vi "lab2_new_p2.vi"() -> ()   [LabVIEW 2021]
panel:
  in  "x":dbl
  out "S":ext
  in  "n":u64
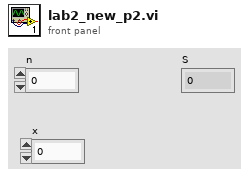
[diagram p1: front panel]
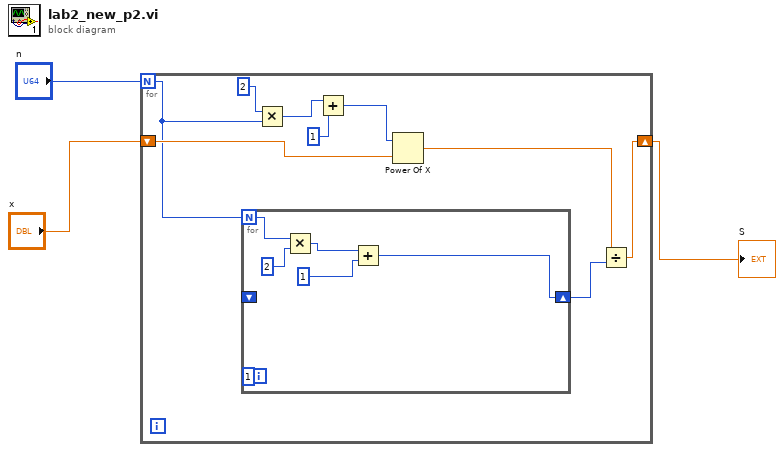
[diagram p0: block diagram]
diagram:
  n1 = for {
    N: "n" -> [w10]
    shift-right: [w4] -> w1
    shift-left: "x" -> [w12]
    n2 = for {
      N: w10 -> [w17]
      shift-right: [w13] -> w5
      shift-left: _ -> [_]
      (unwired) 1
      n3 = Multiply(x=w17, y=2) -> (x*y=w15:i32)
      n4 = Add(x=w15, y=1) -> (x+y=w13:i32)
    }
    n5 = Multiply(x=2, y=w10) -> (x*y=w9:i32)
    n6 = Add(x=w9, y=1) -> (x+y=w7:i32)
    n7 = Power Of X(1:w12, 2:w7) -> (0:w6:dbl)
    n8 = Divide(x=w6, y=w5) -> (x/y=w4:dbl)
  }
  "S" <- w1
